vi "DataStream_init.vi"(4 "buffer size":i32=1, 5 "CTR IP Addr":string="localhost", 6 "timeout ms":i32=-1, 7 "DAQ IP Addr":string="localhost", 8 "error in":errorcluster, 10 "DAQ Endpoint":string="DAQ000", 11 "CTR Endpoint":string="CTR001") -> (0 "error out":errorcluster, 1 "Streams Started?":bool, 2 "reader endpoint":refnum<k21>, 3 "writer endpoint":refnum<k21>)   [LabVIEW 2024]
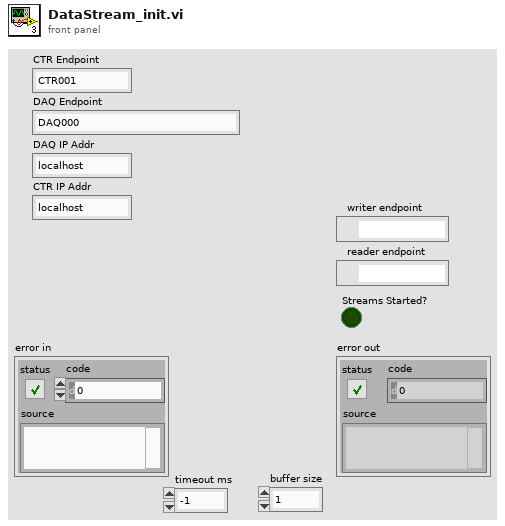
[diagram p1: front panel]
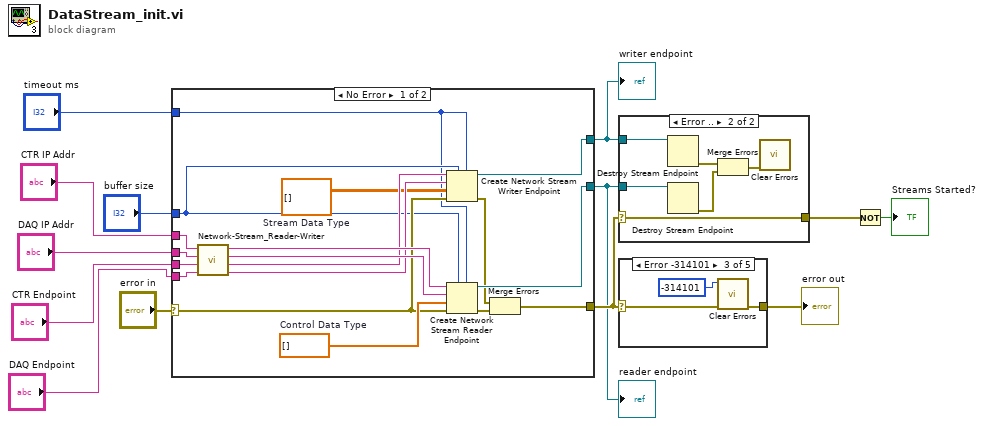
[diagram p0: block diagram]
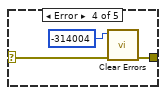
[diagram p5: hidden frame]
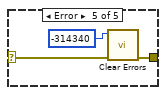
[diagram p6: hidden frame]
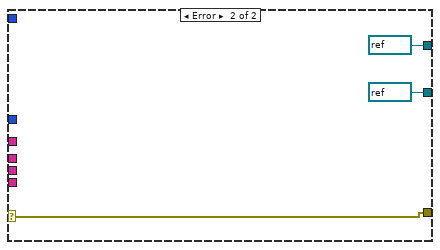
[diagram p7: hidden frame]
diagram:
  n1 = case shown="No Error" "error in" {
    selector: "error in" -> [w19 w34]
    tunnel: [w23 w34] -> w5
    tunnel: [w21 refnum<k21> refnum ("writer endpoint")] -> w2
    tunnel: [w31 refnum<k21> refnum ("reader endpoint")] -> w3
    tunnel: "CTR IP Addr" -> [w29 _]
    tunnel: "DAQ Endpoint" -> [w26 _]
    tunnel: "CTR Endpoint" -> [w27 _]
    tunnel: "DAQ IP Addr" -> [w28 _]
    tunnel: "timeout ms" -> [w14 _]
    tunnel: "buffer size" -> [w15 _]
    frame No Error {
      w16 = dbl[][] []  # Stream Data Type
      w30 = dbl[] []  # Control Data Type
      n2 = call "Network-Stream_Reader-Writer.vi"("DAQ Endpoint"=w26, "CTR Endpoint"=w27, "DAQ IP Addr"=w28, "CTR IP Addr"=w29) -> ("//CTR IP Addr:CTR000/DAQ000-Data"=w17:string, "//DAQ IP Addr:DAQ000/DAQ000-Data"=w18:string, "//CTR IP Addr:CTR000/DAQ000-Control"=w24:string, "//DAQ IP Addr:DAQ000/DAQ000-Control"=w25:string)  [unwired: 4 in]
      n3 = Create Network Stream Writer Endpoint(5:w14, 7:w15, 8:w19, 9:w16, 10:w17, 11:w18) -> (0:w20:errorcluster, 3:w21:refnum<k21>)  [unwired: 1 in]
      n4 = Create Network Stream Reader Endpoint(5:w14, 7:w15, 8:w19, 9:w30, 10:w24, 11:w25) -> (0:w22:errorcluster, 3:w31:refnum<k21>)  [unwired: 1 in]
      n5 = Merge Errors(w20, w22) -> (w23:errorcluster)
    }
    frame Error {
    }
  }
  "writer endpoint" <- w2
  "reader endpoint" <- w3
  n6 = case shown="Error .." w5 {
    selector: w5 -> [w35 w41]
    tunnel: [w35 w41] -> w4
    tunnel: w3 -> [_ w40]
    tunnel: w2 -> [_ w39]
    frame No Error {
    }
    frame Error {
      n7 = Destroy Stream Endpoint(11:w39) -> (0:w37:errorcluster)  [unwired: 1 in]
      n8 = Destroy Stream Endpoint(11:w40) -> (0:w38:errorcluster)  [unwired: 1 in]
      n9 = Merge Errors(w37, w38) -> (w36:errorcluster)
      n10 = call <vilib>:"Clear Errors.vi"("error in (no error)"=w36) -> ()  [unwired: 5 in, 2 out]
    }
  }
  n11 = case shown="Error -314101" w5 {
    selector: w5 -> [w42 w43 w46 w49 w52]
    tunnel: [w42 w43 w45 w48 w51] -> w6
    frame No Error {
    }
    frame Default {
    }
    frame Error {
      n12 = call <vilib>:"Clear Errors.vi"("error in (no error)"=w46, "specific error code to clear (0: all)"=-314101) -> ("error out"=w45:errorcluster)  [unwired: 4 in, 1 out]
    }
    frame Error {
      n13 = call <vilib>:"Clear Errors.vi"("error in (no error)"=w49, "specific error code to clear (0: all)"=-314004) -> ("error out"=w48:errorcluster)  [unwired: 4 in, 1 out]
    }
    frame Error {
      n14 = call <vilib>:"Clear Errors.vi"("error in (no error)"=w52, "specific error code to clear (0: all)"=-314340) -> ("error out"=w51:errorcluster)  [unwired: 4 in, 1 out]
    }
  }
  "error out" <- w6
  n15 = Not(x=w4) -> (.not. x?=→"Streams Started?":bool)
